vi "Scanner Data Position.vi"(8 "error in (no error)":errorcluster, 9 "queue":refnum<queue>, 10 "Scanner notifier":refnum<notifier>, 11 "Hardware Resources in":T1={"Link"={"Connection"=enum."USB", "Host or IP address (TCP/IP)"="", "Port (Serial/USB)"="COM1"}, "VISA resource"="", "Writer Queue"=refnum, "Status"=FALSE}) -> (0 "error out":errorcluster, 2 "Message Data Out":variant, 3 "Hardware Resources out":T1={"Link"={"Connection"=enum."USB", "Host or IP address (TCP/IP)"="", "Port (Serial/USB)"="COM1"}, "VISA resource"="", "Writer Queue"=refnum, "Status"=FALSE})   [LabVIEW 2020, in "Hiden Scanner.lvlib"]
doc: "Generates sample waveforms according to the signal type in the HW Config input."
uses:
  Hiden Scanner.lvlib
  Scanner Hardware Configuration.ctl
  support/Message Queue/Message Cluster.ctl
  <instrlib>/Hiden/Hiden MS.lvlib
  support/Message Queue/Message Queue.lvlib
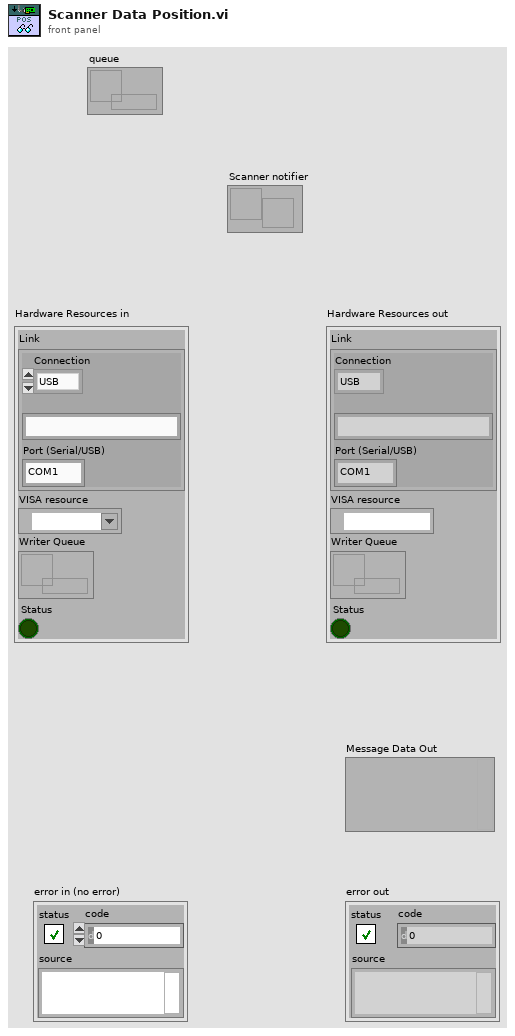
[diagram p1: front panel]
types:
  T1 = typedef "Hiden Scanner.lvlib/Scanner Hardware Configuration.ctl" = cluster{"Link":cluster{"Connection":enum16{"Serial", "TCP/IP", "USB"}, "Host or IP address (TCP/IP)":string, "Port (Serial/USB)":string}, "VISA resource":refnum<visa-resource-name>, "Writer Queue":refnum<queue>, "Status":bool}
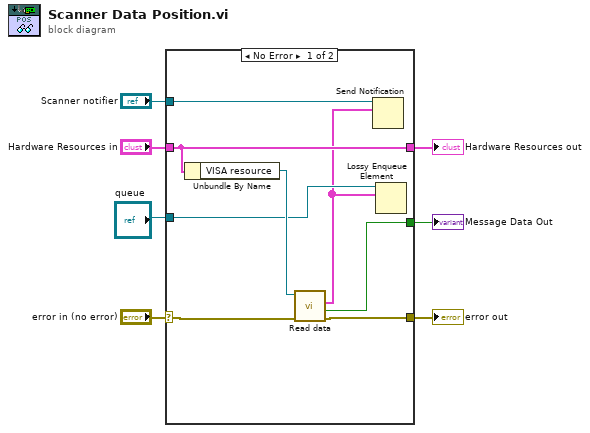
[diagram p0: block diagram]
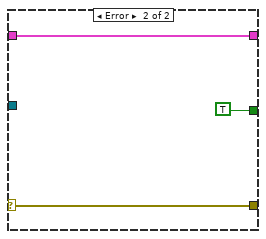
[diagram p2: hidden frame]
diagram:
  n1 = case shown="No Error" "error in (no error)" {
    selector: "error in (no error)" -> [w12 w18]
    tunnel: [w11 w18] -> w6
    tunnel: [w10 TRUE] -> w5
    tunnel: "Hardware Resources in" -> [w14 w17]
    tunnel: [w14 w17] -> w3
    tunnel: "Scanner notifier" -> [w15 _]
    tunnel: "queue" -> [w9 _]
    frame No Error {
      n2 = Unbundle By Name(w14) -> ("VISA resource"=w13:refnum<visa-resource-name>)
      n3 = call <instrlib>:"Read data.vi"("error in (no error)"=w12, "Connection"=w13) -> ("error out"=w11:errorcluster, "Data End?"=w10:bool, "Data out"=w8:cluster{"Timestamp  Stimulus   Value":dbl[][]}[])  [unwired: 6 in, 1 out]
      n4 = Send Notification(notification=w8, notifier=w15) -> ()  [unwired: 1 in, 2 out]
      n5 = Lossy Enqueue Element(queue=w9, element=w8) -> ()  [unwired: 1 in, 4 out]
    }
    frame Error {
    }
  }
  "error out" <- w6
  "Message Data Out" <- w5
  "Hardware Resources out" <- w3
